vi "Periodic Tasks V.5.0.vi"(8 "error in":errorcluster) -> ()   [LabVIEW 2016]
doc: "This VI runs in parallel to other tasks. It can contain as many user-defined periodic loops as you need. These can carry out PID or other sorts of timed response."
uses:
  <vilib>/Rock Robotics/WPI/Utilities/WPI_GetSetVariantRefNum.vi
  Robot Global Data V.5.0.vi
  <vilib>/Rock Robotics/Network Tables/NT Read Boolean.vi
panel:
  out "Gyro":dbl
  out "Back Right":dbl
  out "Back Left":dbl
  out "Front Right":dbl
  out "Front Left":dbl
  # "current values"
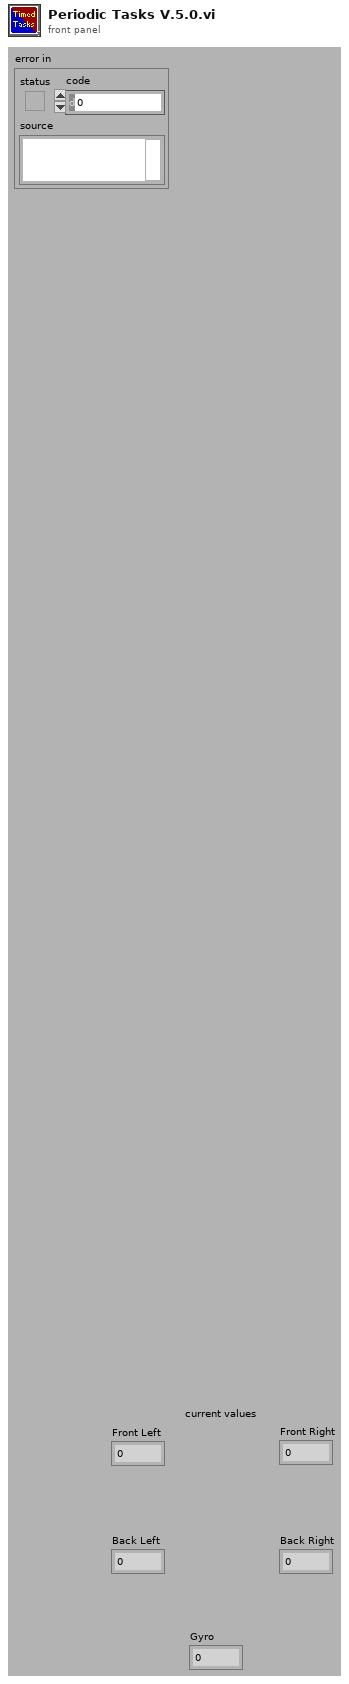
[diagram p1: front panel]
types:
  T1 = typedef "WPI_ServoDeviceRef.ctl" = cluster{"DeviceStatus":errorcluster, "PWM Channel":T2, "DeadBand":T3}
  T2 = typedef "FPGA_DIOPWMChannel.ctl" = enum8{"PWM 0", "PWM 1", "PWM 2", "PWM 3", "PWM 4", "PWM 5", "PWM 6", "PWM 7", "PWM 8", "PWM 9", "PWM MXP 0", "PWM MXP 1", "PWM MXP 2", "PWM MXP 3", "PWM MXP 4", "PWM MXP 5", "PWM MXP 6", "PWM MXP 7", "PWM MXP 8", "PWM MXP 9", "Invalid"}
  T3 = typedef "WPI_PWMDeadband.ctl" = cluster{"Name":string, "maxPositivePwm":i32, "minPositivePwm":i32, "centerPwm":i32, "maxNegativePwm":i32, "minNegativePwm":i32, "angularRange":u16}
  T4 = typedef "WPI_MotorControlDeviceRef.ctl" = cluster{"DeviceStatus":errorcluster, "Type":T5, "PWM":cluster{"PWM Channel":T2, "DeadBand":T3}, "CAN":cluster{"Device Number":u8, "SetOutput VI Ref":variant, "GetOutput VI Ref":variant, "Enable VI Ref":variant, "Disable VI Ref":variant, "Data":variant}, "Invert":bool}
  T5 = typedef "WPI_MotorControlType.ctl" = enum16{"PWM", "CAN"}
  T6 = typedef "WPI_JoystickDevRef.ctl" = cluster{"Device":T7}
  T7 = typedef "WPI_JoystickDeviceEnum.ctl" = enum16{"USB 0", "USB 1", "USB 2", "USB 3", "USB 4", "USB 5"}
  T8 = typedef "WPI_CANTalonSRX_GlobalStatus.ctl" = cluster{"Applied Throttle":dbl, "Module Enabled":bool, "CAN Error":errorcluster, "Closed Loop Error":dbl, "Forward Limit Switch Closed":bool, "Reverse Limit Switch Closed":bool, "Sensor Position":dbl, "Sensor Velocity":dbl, "Current":dbl, "Sticky Fault - Over Temp":bool, "Sticky Fault - Under Voltage":bool, "Sticky Fault - Forward Limit":bool, "Sticky Fault - Reverse Limit":bool, "Sticky Fault - Forward Soft Limit":bool, "Sticky Fault - Reverse Soft Limit":bool, "Brake is Enabled":bool, "Encoder Position":dbl, "Encoder Velocity":dbl, "Encoder Index Count":dbl, "Encoder A Pin State":bool, "Encoder B Pin State":bool, "Encoder Index Pin State":bool, "Analog In":dbl, "Analog In Velocity":dbl, "Temperature (C)":dbl, "Battery Voltage":dbl, "Control 5 Is Supported":bool, "Current Profile Slot Select":dbl, "Pos Div 8":bool, "Vel Div 4":bool, "Pulse Width Position":i32, "Pulse Width Velocity":i32, "Pulse Width Rise To Rise (us)":i32, "Pulse Width Rise To Fall (us)":i32, "Mot Prof Active Is Under Run":bool, "Mot Prof Active Has Under Run":bool, "Mot Prof Active Is Last":bool, "Mot Prof Active Velocity Only":bool, "Mot Prof Active Is Valid":bool, "Mot Prof Buffer Is Full":bool, "Mot Prof Active Profile Slot Select":i32, "Mot Prof NextID":i32, "Mot Prof Count":i32, "Mot Prof Active Velocity":dbl, "Mot Prof Active Position":dbl, "Mot Prof Output Enable":i32}
  T9 = typedef "WPI_RobotDriveDevRef.ctl" = cluster{"DevStatus":errorcluster, "Motors[]":T4[], "Square Inputs":bool, "Max Output":dbl}
  T10 = typedef "WPI_CompressorDevRef.ctl" = cluster{"DevStatus":errorcluster, "Pneumatics Control Module":u8}
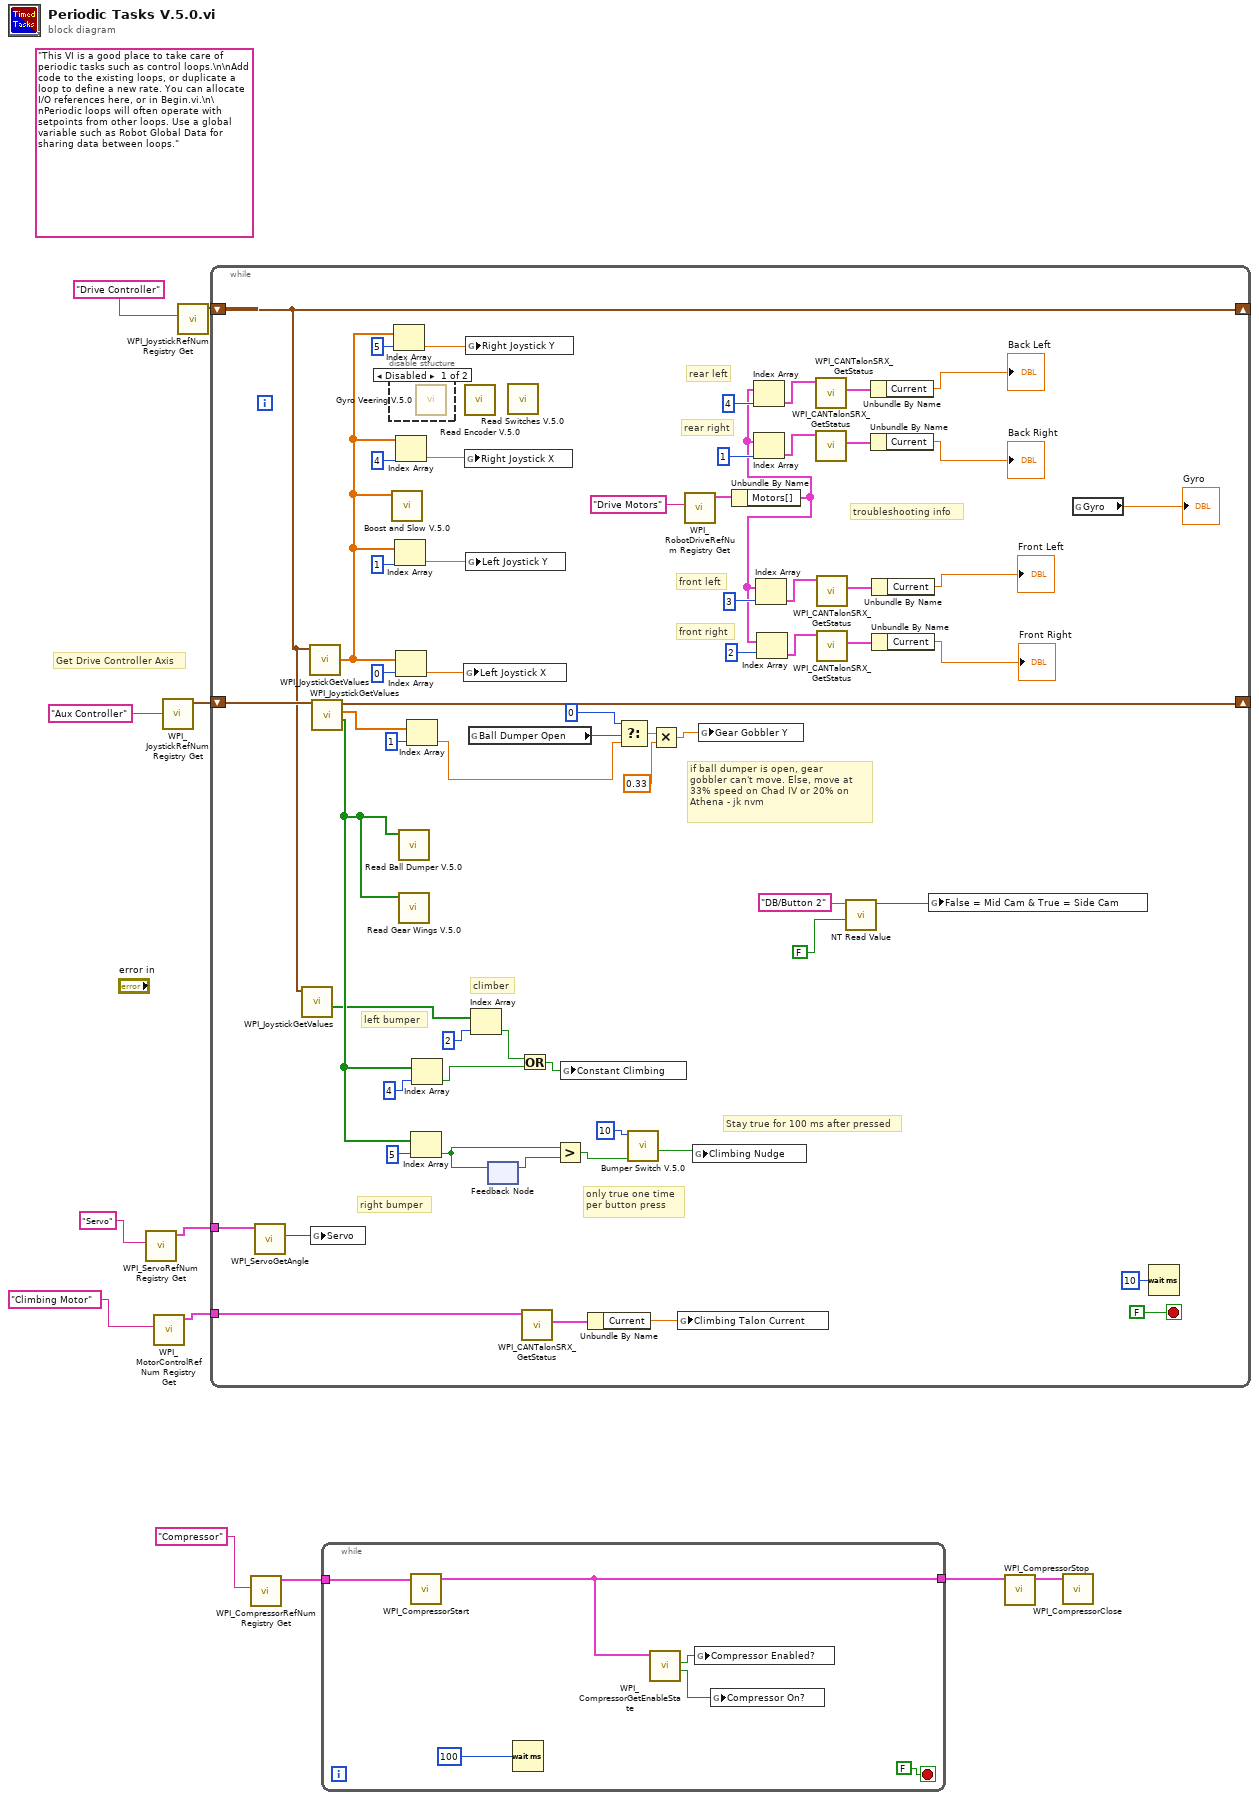
[diagram p0: block diagram]
diagram:
  (unwired) "This VI is a good place to take care of periodic tasks such as control loops.\n\nAdd code to the existing loops, or duplicate a loop to define a new rate. You can allocate I/O references here, or in Begin.vi.\n\nPeriodic loops will often operate with setpoints from other loops. Use a global variable such as Robot Global Data for sharing data between loops."
  # "Get Drive Controller Axis"
  n1 = call <vilib>:"WPI_ServoRefNum Registry Get.vi"("refnum name"="Servo") -> ("ServoDeviceRef"=w2:T1)  [unwired: 9 in, 1 out]
  n2 = call <vilib>:"WPI_MotorControlRefNum Registry Get.vi"("refnum name"="Climbing Motor") -> ("MotorControlDevRef"=w3:T4)  [unwired: 9 in, 1 out]
  n3 = call <vilib>:"WPI_JoystickRefNum Registry Get.vi"("refnum name"="Aux Controller") -> ("JoystickDevRef"=w9:T6)  [unwired: 1 in, 9 out]
  n4 = call <vilib>:"WPI_JoystickRefNum Registry Get.vi"("refnum name"="Drive Controller") -> ("JoystickDevRef"=w11:T6)  [unwired: 1 in, 9 out]
  n5 = while {
    shift-right: [w14] -> _
    shift-left: w11 -> [w14]
    shift-right: [w66] -> _
    shift-left: w9 -> [w67]
    tunnel: w3 -> [w44]
    tunnel: w2 -> [w43]
    stop <- FALSE stop-if-true
    # "troubleshooting info"
    # "front right"
    # "front left"
    # "rear right"
    # "rear left"
    # "Stay true for 100 ms after pressed"
    # "only true one time\nper button press"
    # "right bumper"
    # "left bumper"
    # "if ball dumper is open, gear \ngobbler can't move. Else, move at \n33% speed on Chad IV or 20% on \nAthena - jk nvm"
    # "climber"
    n6 = call <vilib>:"WPI_ServoGetAngle.vi"("ServoDeviceRef"=w43) -> ("Angle"=w42:u16)  [unwired: 7 in, 2 out]
    n7 = call <vilib>:"WPI_JoystickGetValues.vi"("JoystickDevRef"=w14) -> ("Buttons"=w13:bool[])  [unwired: 6 in, 4 out]
    n8 = call <vilib>:"WPI_JoystickGetValues.vi"("JoystickDevRef"=w14) -> ("Axes"=w46:dbl[])  [unwired: 6 in, 4 out]
    n9 = global write "Robot Global Data V.5.0.vi" "Servo"(w42) -> ()
    n10 = call <vilib>:"WPI_JoystickGetValues.vi"("JoystickDevRef"=w67) -> ("Buttons"=w45:bool[], "Axes"=w54:dbl[], "JoystickDevRef"=w66:T6)  [unwired: 6 in, 2 out]
    n11 = disable-structure shown="Disabled" {
      frame Disabled {
        n12 = call "Gyro Veering V.5.0.vi"() -> ()  [unwired: 12 in]
      }
      frame Enabled {
      }
    }
    n13 = call "Boost and Slow V.5.0.vi"("Drive Axises"=w46) -> ()  [unwired: 11 in]
    n14 = Index Array(array=w46, index=5) -> (element=w65:dbl)
    n15 = Index Array(array=w46, index=1) -> (element=w64:dbl)
    n16 = Index Array(array=w46, index=4) -> (element=w72:dbl)
    n17 = Index Array(array=w46, index=0) -> (element=w73:dbl)
    n18 = call "Read Ball Dumper V.5.0.vi"("Joystick Buttons"=w45) -> ()  [unwired: 11 in]
    n19 = call "Read Gear Wings V.5.0.vi"("Joystick Buttons"=w45) -> ()  [unwired: 11 in]
    n20 = Index Array(array=w54, index=1) -> (element=w51:dbl)
    n21 = Index Array(array=w45, index=5) -> (element=w59:bool)
    n22 = Index Array(array=w45, index=4) -> (element=w16:bool)
    n23 = global write "Robot Global Data V.5.0.vi" "Left Joystick X"(w73) -> ()
    n24 = call "Read Encoder V.5.0.vi"() -> ()  [unwired: 12 in]
    n25 = global write "Robot Global Data V.5.0.vi" "Right Joystick X"(w72) -> ()
    n26 = global write "Robot Global Data V.5.0.vi" "Right Joystick Y"(w65) -> ()
    n27 = global write "Robot Global Data V.5.0.vi" "Left Joystick Y"(w64) -> ()
    n28 = global read "Robot Global Data V.5.0.vi" "Ball Dumper Open"() -> (w52:bool)
    n29 = Index Array(array=w13, index=2) -> (element=w17:bool)
    n30 = feedback-in #1(w59) -> ()
    n31 = feedback #1() -> (w60:bool)  [unwired: 1 in]
    n32 = call "Read Switches V.5.0.vi"() -> ()  [unwired: 12 in]
    n33 = Or(x=w17, y=w16) -> (x .or. y?=w15:bool)
    n34 = call <vilib>:"WPI_CANTalonSRX_GetStatus.vi"("CAN Talon SRX Ref"=w44) -> ("Talon SRX Status"=w63:T8)  [unwired: 8 in, 2 out]
    n35 = Greater?(x=w59, y=w60) -> (0:w58:bool)
    n36 = global write "Robot Global Data V.5.0.vi" "Constant Climbing"(w15) -> ()
    n37 = Unbundle By Name(w63) -> ("Current"=w62:dbl)
    n38 = Select(t=0, s=w52, f=w51) -> (s? t:f=w49:dbl)
    n39 = call "Bumper Switch V.5.0.vi"("Input Button"=w58, "TIme until Reset"=10) -> ("On?"=w55:bool)  [unwired: 9 in]
    n40 = Multiply(x=w49, y=0.33) -> (x*y=w48:dbl)
    n41 = global write "Robot Global Data V.5.0.vi" "Climbing Talon Current"(w62) -> ()
    n42 = call <vilib>:"WPI_RobotDriveRefNum Registry Get.vi"("refnum name"="Drive Motors") -> ("RobotDriveDevRef"=w40:T9)  [unwired: 9 in, 1 out]
    n43 = global write "Robot Global Data V.5.0.vi" "Climbing Nudge"(w55) -> ()
    n44 = global write "Robot Global Data V.5.0.vi" "Gear Gobbler Y"(w48) -> ()
    n45 = Unbundle By Name(w40) -> ("Motors[]"=w35:T4[])
    n46 = Index Array(array=w35, index=4) -> (element=w34:T4)
    n47 = Index Array(array=w35, index=1) -> (element=w29:T4)
    n48 = Index Array(array=w35, index=3) -> (element=w28:T4)
    n49 = Index Array(array=w35, index=2) -> (element=w22:T4)
    n50 = call <vilib>:"WPI_CANTalonSRX_GetStatus.vi"("CAN Talon SRX Ref"=w34) -> ("Talon SRX Status"=w33:T8)  [unwired: 8 in, 2 out]
    n51 = call <vilib>:"WPI_CANTalonSRX_GetStatus.vi"("CAN Talon SRX Ref"=w29) -> ("Talon SRX Status"=w32:T8)  [unwired: 8 in, 2 out]
    n52 = call <vilib>:"WPI_CANTalonSRX_GetStatus.vi"("CAN Talon SRX Ref"=w28) -> ("Talon SRX Status"=w31:T8)  [unwired: 8 in, 2 out]
    n53 = call <vilib>:"WPI_CANTalonSRX_GetStatus.vi"("CAN Talon SRX Ref"=w22) -> ("Talon SRX Status"=w30:T8)  [unwired: 8 in, 2 out]
    n54 = call-poly <vilib>:"NT Read Value.vi"("Default Value"=FALSE, "Name"="DB/Button 2" ("refnum name")) -> ("Boolean"=w20:bool)  [unwired: 8 in, 1 out]
    n55 = Unbundle By Name(w33) -> ("Current"=→"Back Left":dbl)
    n56 = Unbundle By Name(w32) -> ("Current"=→"Back Right":dbl)
    n57 = Unbundle By Name(w31) -> ("Current"=→"Front Left":dbl)
    n58 = Unbundle By Name(w30) -> ("Current"=→"Front Right":dbl)
    n59 = global write "Robot Global Data V.5.0.vi" "False = Mid Cam & True = Side Cam"(w20) -> ()
    n60 = global read "Robot Global Data V.5.0.vi" "Gyro"() -> (→"Gyro":dbl)
    n61 = Wait (ms)(milliseconds to wait=u32 10) -> ()  [unwired: 1 out]
  }
  n62 = call <vilib>:"WPI_CompressorRefNum Registry Get.vi"("refnum name"="Compressor") -> ("CompressorDevRef"=w8:T10)  [unwired: 9 in, 1 out]
  n63 = while {
    tunnel: w8 -> [w80]
    tunnel: [w78] -> w6
    stop <- FALSE stop-if-true
    n64 = call <vilib>:"WPI_CompressorStart.vi"("CompressorDevRef"=w80) -> ("CompressorDevRef"=w78:T10)  [unwired: 9 in, 1 out]
    n65 = Wait (ms)(milliseconds to wait=100) -> ()  [unwired: 1 out]
    n66 = call <vilib>:"WPI_CompressorGetEnableState.vi"("CompressorDevRef"=w78) -> ("Compressor Running"=w76:bool, "Enabled"=w77:bool)  [unwired: 7 in, 2 out]
    n67 = global write "Robot Global Data V.5.0.vi" "Compressor Enabled?"(w77) -> ()
    n68 = global write "Robot Global Data V.5.0.vi" "Compressor On?"(w76) -> ()
  }
  n69 = call <vilib>:"WPI_CompressorStop.vi"("CompressorDevRef"=w6) -> ("CompressorDevRef"=w5:T10)  [unwired: 9 in, 1 out]
  n70 = call <vilib>:"WPI_CompressorClose.vi"("CompressorDevRef"=w5) -> ()  [unwired: 10 in, 1 out]
